vi "Close.vi"(8 "error in (no error)":errorcluster, 11 "PreUUT in":refnum<class "PreUUT.lvclass">) -> (0 "error out":errorcluster, 3 "PreUUT out":refnum<class "PreUUT.lvclass">)   [LabVIEW 2019, in "Sequence Main.lvlib" / "PreUUT.lvclass"]
uses:
  PreUUT.lvclass
  PreUUT.lvclass/PreUUT.ctl
  Abstract UUT/Abstract UUT.lvclass
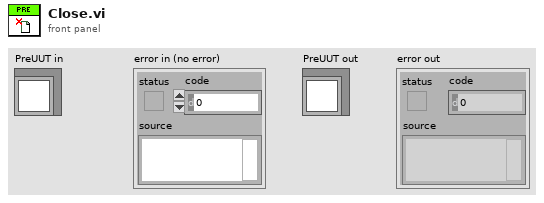
[diagram p1: front panel]
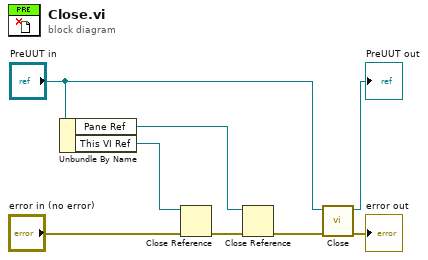
[diagram p0: block diagram]
diagram:
  n1 = Unbundle By Name("PreUUT in") -> ("Pane Ref"=w2:refnum<vi>, "This VI Ref"=w5:refnum<vi>)
  n2 = Close Reference(reference=w5, error in (no error)="error in (no error)") -> (error out=w3:errorcluster)
  n3 = Close Reference(reference=w2, error in (no error)=w3) -> (error out=w1:errorcluster)
  n4 = call-parent "Close.vi"("error in (no error)"=w1, "Abstract UUT in"="PreUUT in") -> ("error out"=→"error out":errorcluster, "Abstract UUT out"=→"PreUUT out":refnum<class "PreUUT.lvclass">)  [unwired: 8 in]
